vi "Get Module Execution Status by ref.vi"(6 "Modules Tree ref":refnum<vi>, 11 "Refs":T1) -> (0 "error out":errorcluster)   [LabVIEW 2019, in "Panther Dashboard.lvlib"]
doc: "This VI checks the Main.vi State of the selected DQMH Module"
uses:
  Panther Dashboard.lvlib
  References Updated Argument--cluster.ctl
  Module type--enum.ctl
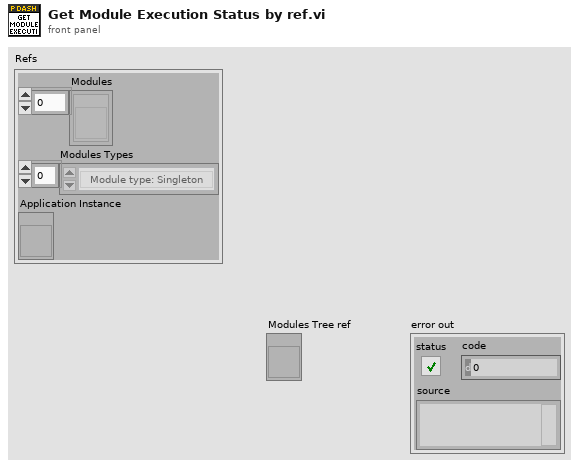
[diagram p1: front panel]
types:
  T1 = typedef "Panther Dashboard.lvlib/References Updated Argument--cluster.ctl" = cluster{"Modules":refnum<vi>[], "Modules Types":T2[], "Application Instance":refnum<vi>}
  T2 = typedef "Panther Dashboard.lvlib/Module type--enum.ctl" = enum16{"Module type: Singleton", "Module type: Cloneable"}
  T3 = enum32{"Bad", "Idle", "Run top level", "Running"}
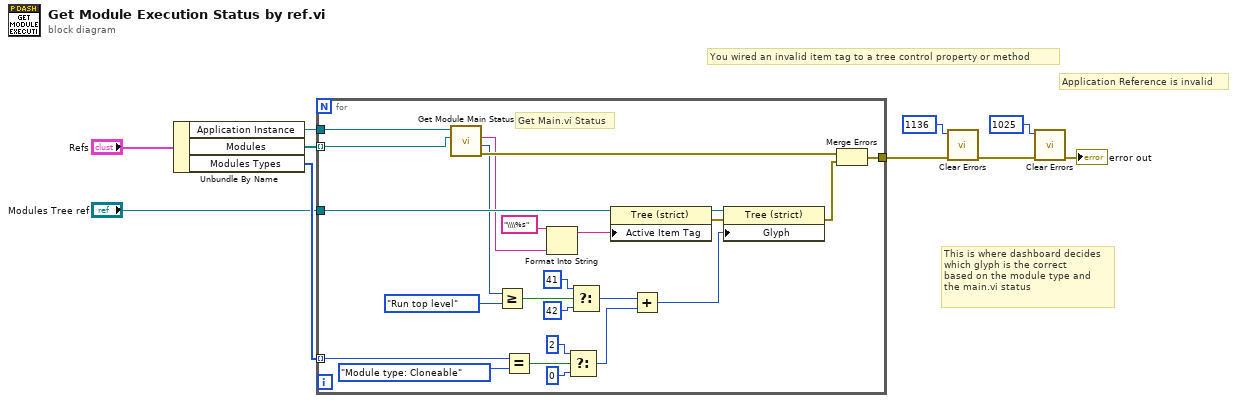
[diagram p0: block diagram]
diagram:
  # "This is where dashboard decides\nwhich glyph is the correct\nbased on the module type and\nthe main.vi status"
  # "Application Reference is invalid"
  # "You wired an invalid item tag to a tree control property or method"
  n1 = Unbundle By Name("Refs") -> ("Application Instance"=w5:refnum<vi>, "Modules"=w4:refnum<vi>[], "Modules Types"=w3:T2[])
  n2 = for {
    tunnel: [w33] -> w10
    tunnel: w4 -> [w12] mode=indexing
    tunnel: "Modules Tree ref" -> [w29]
    tunnel: w3 -> [w20] mode=indexing
    tunnel: w5 -> [w13]
    # "Get Main.vi Status"
    n3 = call "Get Module Main Status.vi"("Library in"=w12, "application Instance"=w13) -> ("error out"=w31:errorcluster, "Module Exec State"=w11:T3, "Library Name"=w14:string)  [unwired: 7 in]
    n4 = Greater Or Equal?(x=w11, y=T3."Run top level") -> (x >= y?=w24:bool)
    n5 = Equal?(x=w20, y=Module_type--enum."Module type: Cloneable" ("x")) -> (x = y?=w18:bool)
    n6 = Format Into String(format string="\\\\%s", w14) -> (resulting string=w28:string)  [unwired: 2 in, 1 out]
    n7 = Select(t=2, s=w18, f=0) -> (s? t:f=w15:i32)
    n8 = Select(t=41, s=w24, f=42) -> (s? t:f=w26:i32)
    n9 = property class="Tree (strict)"(reference=w29, "Active Item Tag"=w28) -> (reference out=w27:refnum<vi>, error out=w34:errorcluster)  [unwired: 1 in]
    n10 = Add(x=w26, y=w15) -> (x+y=w21:i32)
    n11 = property class="Tree (strict)"(reference=w27, error in=w34, "Glyph"=w21) -> (error out=w32:errorcluster)  [unwired: 1 out]
    n12 = Merge Errors(w31, w32) -> (w33:errorcluster)
  }
  n13 = call <vilib>:"Clear Errors.vi"("error in (no error)"=w10, "specific error code to clear (0: all)"=1136) -> ("error out"=w9:errorcluster)  [unwired: 4 in, 1 out]
  n14 = call <vilib>:"Clear Errors.vi"("error in (no error)"=w9, "specific error code to clear (0: all)"=1025) -> ("error out"=→"error out":errorcluster)  [unwired: 4 in, 1 out]
